vi "Cross product 2D.vi"(1 "B":sgl[](array[numeric])=[0.0, 0.0], 2 "A":sgl[](array[numeric])=[0.0, 0.0]) -> (0 "A X B":sgl)   [LabVIEW 2014]
panel:
  # "PN 12/01/2015"
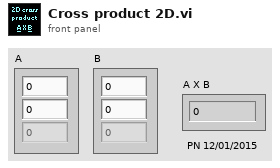
[diagram p1: front panel]
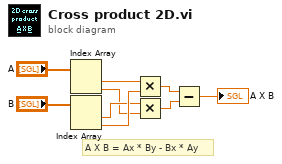
[diagram p0: block diagram]
diagram:
  # "A X B = Ax * By - Bx * Ay"
  n1 = Index Array(array="A") -> (element #1=w4:sgl, element #2=w1:sgl)  [unwired: 2 in]
  n2 = Index Array(array="B") -> (element #1=w2:sgl, element #2=w3:sgl)  [unwired: 2 in]
  n3 = Multiply(x=w4, y=w3) -> (x*y=w6:sgl)
  n4 = Multiply(x=w2, y=w1) -> (x*y=w7:sgl)
  n5 = Subtract(x=w6, y=w7) -> (x-y=→"A X B":sgl)
